vi "is abstract node.vi"(8 "error in":errorcluster, 11 "fixed channel editor in":refnum<class "fixed channel editor.lvclass">) -> (0 "error out":errorcluster, 2 "abstract":bool, 3 "fixed channel editor out":refnum<class "fixed channel editor.lvclass">)   [LabVIEW 2013, in "fixed channel editor.lvclass"]
uses:
  fixed channel editor.lvclass
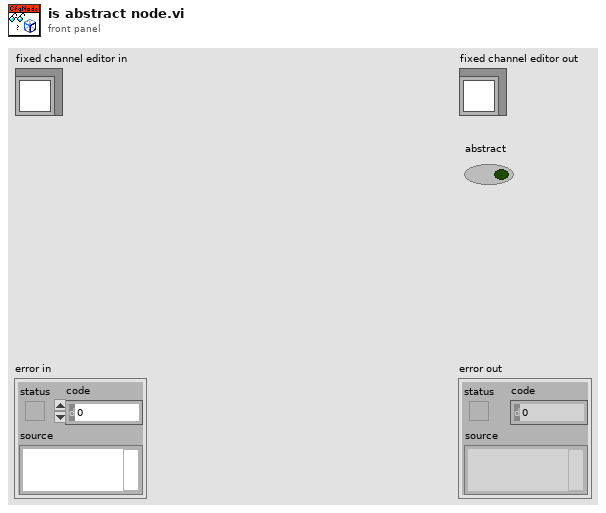
[diagram p1: front panel]
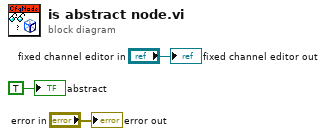
[diagram p0: block diagram]
diagram:
  "error out" <- "error in"
  "fixed channel editor out" <- "fixed channel editor in"
  "abstract" <- TRUE ("abstract")
